vi "列表框拖动与放置(移动).vi"() -> ()   [LabVIEW 2012, in "Listbox Tool.lvlib"]
uses:
  Listbox Tool.lvlib
  Custom Type/Drag and Drop.ctl
  Custom Type/Read and Write Mode.ctl
  Property/Drag and Drop.vi
panel:
  in  "水浒人物":i32[](listbox)
  in  "停止":bool
  in  "三国人物":i32[](listbox)
  in  "西游记人物":i32[](listbox)
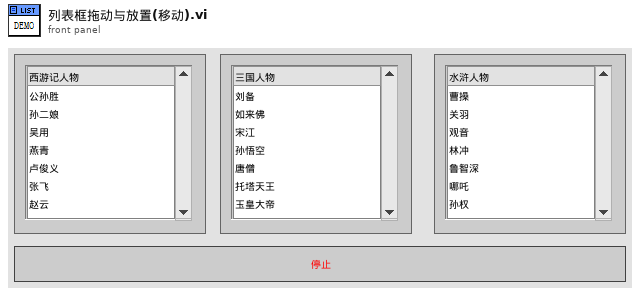
[diagram p1: front panel]
types:
  T1 = typedef "Listbox Tool.lvlib/Drag and Drop.ctl" = cluster{"拖曳/放置:拖曳模式":enum32{"copy or move", "copy only", "move only"}, "拖曳/放置:允许拖曳":bool, "拖曳/放置:允许放置":bool, "拖曳/放置:允许拖曳和放置外部控件":bool}
  T2 = typedef "Listbox Tool.lvlib/Read and Write Mode.ctl" = enum16{"Read", "Write"}
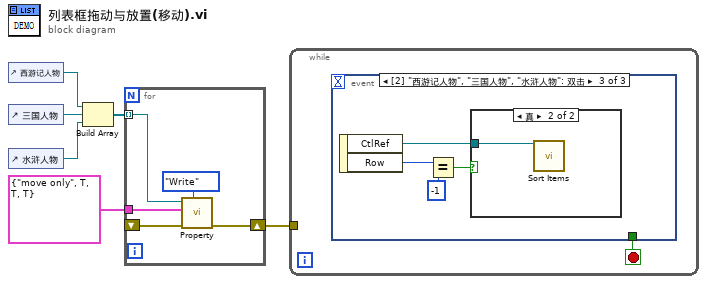
[diagram p0: block diagram]
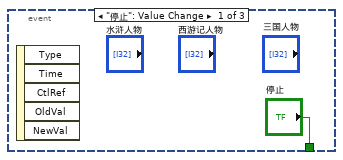
[diagram p2: hidden frame]
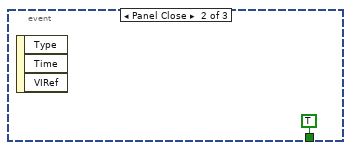
[diagram p3: hidden frame]
diagram:
  n1 = control-ref of="西游记人物"() -> (w6:refnum<vi>)
  n2 = control-ref of="三国人物"() -> (w5:refnum<vi>)
  n3 = control-ref of="水浒人物"() -> (w4:refnum<vi>)
  n4 = Build Array(w6, w5, w4) -> (w3:refnum<vi>[])
  n5 = for {
    tunnel: w3 -> [w11] mode=indexing
    tunnel: T1 {"拖曳/放置:拖曳模式"=enum."move only", "拖曳/放置:允许拖曳"=TRUE, "拖曳/放置:允许放置"=TRUE, "拖曳/放置:允许拖曳和放置外部控件"=TRUE} ("Drag and Drop In") -> [w9]
    shift-right: [w8] -> w1
    shift-left: _ -> [w7]
    n6 = call-poly "Property.vi"("Mode"=Read_and_Write_Mode."Write", "错误输入"=w7, "Drag and Drop In"=w9, "Listbox Ref"=w11) -> ("错误输出"=w8:errorcluster)  [unwired: 5 in, 2 out]
  }
  n7 = while {
    tunnel: w1 -> [_]
    stop <- w12 stop-if-true
    n8 = event shown="[2] \"西游记人物\", \"三国人物\", \"水浒人物\": 双击" {
      selector: _ -> [_ _ _]
      dyn-events: _ -> [_ _ _]
      timeout: _ -> [_ _ _]
      tunnel: ["停止" TRUE ("停止") _] -> w12
      event "停止": Value Change {
        n9 = event-data() -> ()  [unwired: 1 in, 5 out]
      }
      event Panel Close {
        n10 = event-data() -> ()  [unwired: 1 in, 3 out]
      }
      event "西游记人物", "三国人物", "水浒人物": Double Click {
        n11 = event-data() -> ("CtlRef"=w15:refnum<vi>, "Row"=w18:i32)  [unwired: 1 in]
        n12 = Equal?(x=w18, y=-1) -> (x = y?=w16:bool)
        n13 = case shown="真" w16 {
          tunnel: w15 -> [_ w19]
          frame False {
          }
          frame True {
            n14 = call "Sort Items.vi"("Listbox Ref"=w19) -> ()  [unwired: 9 in, 2 out]
          }
        }
      }
    }
  }
